vi "Pre Initialize Config.vi"(8 "error in (no error)":errorcluster, 10 "Pre Initialization Data":variant, 11 "Instrument in":refnum<class "Instrument Driver.lvclass">) -> (0 "error out":errorcluster, 1 "Success?":bool, 3 "Instrument out":refnum<class "Instrument Driver.lvclass">)   [LabVIEW 2020, in "Instrument Driver.lvlib" / "Instrument Driver.lvclass"]
doc: "Populate and configure the Instrument Private data before Initalize using children implementations of this VI.\n\nThe default implementation does nothing."
uses:
  Instrument Driver.lvclass
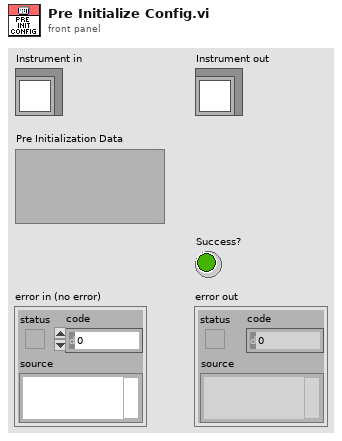
[diagram p1: front panel]
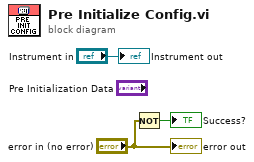
[diagram p0: block diagram]
diagram:
  n1 = Not(x="error in (no error)") -> (.not. x?=→"Success?":bool)
  "error out" <- "error in (no error)"
  "Instrument out" <- "Instrument in"
